vi "Get Calibration State.vi"(8 "error in":errorcluster, 11 "Calibration UI in":refnum<class "Calibration UI.lvclass">) -> (0 "error out":errorcluster, 2 "Action":u32, 3 "Calibration UI out":refnum<class "Calibration UI.lvclass">)   [LabVIEW 2015, in "Calibration UI.lvclass"]
doc: "Retrieve the notifier calibration state. The <b>Action</b> property is determined by the conversion of three bits to a U32. The three bits are: 1) Current calibration state; 2) Notifier wait state; and 3) Notifier availability.The action will tell the caller what the current state is. The actions are as follows:\n* 0: No timeout; stop calibration\n* 1: No timeout; start calibration\n* 2: Timeout; no active calibration\n* 3: Timeout; active calibration\n* > 4: Notifier not available - shutdown\n\nIf the current state is 0 or 2, then the the wait on the notifier will be set to -1 (wait indefinitely). If a calibration is active (1 or 3), then the wait on the notifier is set to 0."
uses:
  Calibration UI.lvclass
  Calibration UI.lvclass/Calibration UI.ctl
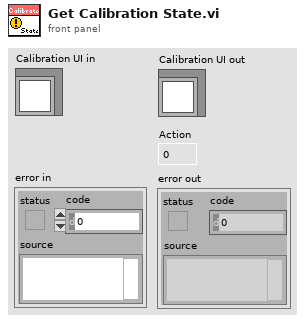
[diagram p1: front panel]
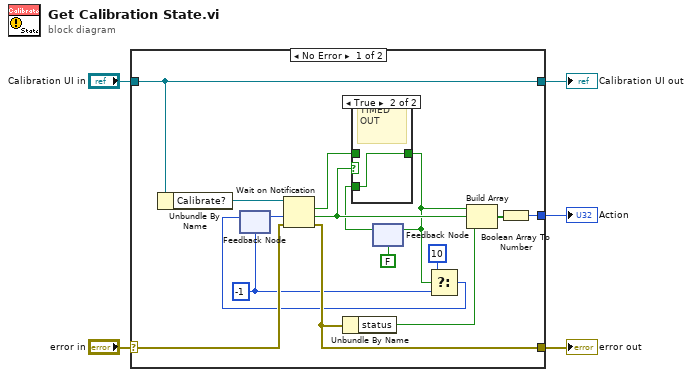
[diagram p0: block diagram]
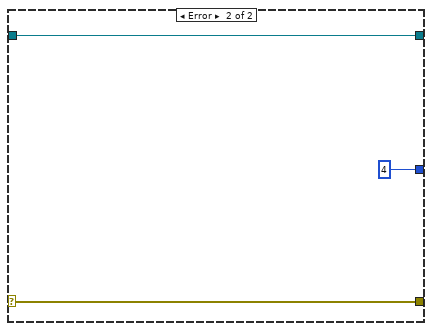
[diagram p3: hidden frame]
diagram:
  n1 = case shown="No Error" "error in" {
    selector: "error in" -> [w14 w26]
    tunnel: [w13 w26] -> w4
    tunnel: [w21 w25] -> w2
    tunnel: "Calibration UI in" -> [w21 w25]
    tunnel: [w17 u32 4] -> w1
    frame No Error {
      w11 = -1 ("timeout in ms (-1)")
      n2 = Unbundle By Name(w21) -> ("Calibrate?"=w20:refnum<notifier>)
      n3 = feedback #1(w11) -> (w16:i32)
      n4 = Wait on Notification(notifier=w20, timeout in ms (-1)=w16, error in (no error)=w14) -> (notification=w9:bool, timed out?=w10:bool, error out=w13:errorcluster)  [unwired: 1 in, 1 out]
      n5 = Unbundle By Name(w13) -> ("status"=w19:bool)
      n6 = feedback #2(FALSE ("timed out?")) -> (w8:bool)
      n7 = case shown="True" w10 {
        tunnel: w9 -> [w22 _]
        tunnel: [w22 w23] -> w6
        tunnel: w8 -> [_ w23]
        frame False {
          # "NEW\nDATA"
        }
        frame True {
          # "TIMED \nOUT"
        }
      }
      n8 = feedback-in #2(w6) -> ()
      n9 = Select(t=10, s=w6, f=w11) -> (s? t:f=w12:i32)
      n10 = feedback-in #1(w12) -> ()
      n11 = Build Array(w6, w10, w19) -> (w18:bool[])
      n12 = Boolean Array To Number(Boolean array=w18) -> (number=w17:u32)
    }
    frame Error {
    }
  }
  "error out" <- w4
  "Calibration UI out" <- w2
  "Action" <- w1
